vi "RT Driver VI.vi"(7 "Operation":T1, 11 "Device Reference in":T2 format="%.0x") -> (0 "Error Code":i32)   [LabVIEW 2015, in "Fuel Injection Addon Engine.lvlib"]
uses:
  Fuel Injection Addon Engine.lvlib
  <vilib>/NI Veristand/Custom Device API/Custom Device Item Ref.ctl
  <vilib>/NI Veristand/Custom Device API/Hardware Interface Driver VI Operation.ctl
  Shared/Types/Compiled.Settings.ctl
  Shared/Types/Injector info.ctl
  <vilib>/NI Veristand/Custom Device API/Waveform Data Reference.ctl
  <vilib>/NI Veristand/Custom Device API/Block Data Reference.ctl
  <vilib>/NI Veristand/Custom Device API/Data Reference.ctl
  Shared/Types/VS.Register.Info.ctl
  Shared/Types/Register.Info.ctl
  Shared/Types/FPGA Data Types.ctl
  Shared/Types/Analysis.Channels.Select.ctl
  Shared/Types/Shot.Parameters.ctl
  Shared/Types/Stage.Parameters.ctl
  Shared/Types/Stage.PullIn.Types.ctl
  Shared/Types/Stage.Transition.Types.ctl
  <vilib>/NI/NIVS Inline Async API/_VS Inline Async API/VS Inline Async API/VS Inline Async API.lvclass/VS Inline Async API.ctl
  <vilib>/NI/NIVS Inline Async API/_Data Access Engine/Data Access Engine/Data Access Engine.lvclass/Data Access Engine.ctl
  <vilib>/NI/NIVS Inline Async API/_Data Access Engine/Access Type Classes/Write/Write.lvclass/Write.ctl
  <vilib>/NI/NIVS Inline Async API/_Data Access Engine/Access Type Classes/ReadWrite/ReadWrite.lvclass/ReadWrite.ctl
  <vilib>/NI/NIVS Inline Async API/_Data Access Engine/Access Type Classes/Read/Read.lvclass/Read.ctl
  <vilib>/NI/NIVS Inline Async API/_Data Access Engine/Data Access Engine/Methods/Data.Engine.Read Data from HW.vi
  <vilib>/NI/NIVS Inline Async API/_VS Inline Async API/Error Handling Process/SubVIs/Error.GetError.vi
  <vilib>/NI/NIVS Inline Async API/_Data Access Engine/Data Access Engine/Methods/Data.Engine.Write Data to HW.vi
  <vilib>/NI/NIVS Inline Async API/_Data Access Engine/Access Type Classes/ReadWrite/ReadWrite.EngineData.vi
  <vilib>/NI/NIVS Inline Async API/_Data Access Engine/Access Type Classes/Write/Write.EngineData.vi
  <vilib>/NI/NIVS Inline Async API/_Data Access Engine/Access Type Classes/Read/Read.EngineData.vi
  <vilib>/NI Veristand/Custom Device API/NI VeriStand - Get Channel Value by Data Reference.vi
  <vilib>/NI Veristand/Custom Device API/NI VeriStand - Set Channel Value by Data Reference.vi
  <vilib>/FPGAPlugInAG/Dynamic/niLvFpga_Close_Dynamic.vi
  <vilib>/NI Veristand/Custom Device API/Global Data Refs.vi
  <vilib>/Utility/error.llb/Error Cluster From Error Code.vi
  <vilib>/rvi/errors/niLvFpgaAdjustHostInterfaceError.vi
  <vilib>/RVI Host/nirviSupport.llb/nirviErrorClusterFromErrorCode.vi
  <vilib>/Utility/config.llb/Close Config Data.vi
  <vilib>/Utility/config.llb/Write Key.vi
  <vilib>/Utility/config.llb/Write Key (I32).vi
  <vilib>/Utility/config.llb/Get Key Names.vi
  <vilib>/Utility/config.llb/Open Config Data.vi
  <vilib>/NI Veristand/Custom Device API/Get Item Property (Variant).vi
  Shared/Constants.vi
  <vilib>/rvi/interface/nirviCloseFPGA/nirviCloseFPGA.xnode
  <vilib>/rvi/interface/nirviMethod/nirviMethod.xnode
  <vilib>/NI Veristand/Custom Device Tools/Custom Device Utility Library/Custom Device Utility Library.lvlib
  <vilib>/NI/NIVS Inline Async API/_VS Inline Async API/VS Inline Async API/VS Inline Async API.lvclass
  <vilib>/rvi/interface/nirviMethod/StockFPGA_InlinedMethodWaitForSingleIRQ.vi
  <vilib>/FPGAPlugInAG/Dynamic/niLvFpga_WaitOnIrq_Dynamic.vi
  <vilib>/FPGAPlugInAG/Dynamic/niLvFpga_AcknowledgeIrq_Dynamic.vi
  <vilib>/NI VeriStand/Custom Device API/Custom Device API.lvlib
  Shared/Fuel Injection Addon Shared.lvlib
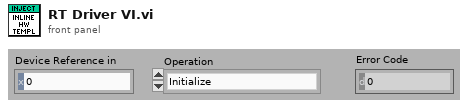
[diagram p1: front panel]
types:
  T1 = typedef "Custom Device API.lvlib/Hardware Interface Driver VI Operation.ctl" = enum16{"Initialize", "Start", "Read Data from HW", "Write Data to HW", "Close"}
  T2 = typedef "Custom Device API.lvlib/Custom Device Item Ref.ctl" = u64
  T3 = typedef "Fuel Injection Addon Engine.lvlib/Inline State Data.ctl" = cluster{"FPGA Ref":refnum<k20>, "Inline Error":errorcluster, "Sample rate (Hz)":u32, "Async":refnum<class "VS Inline Async API.lvclass">, "FPGA.Registers":T4[], "VS.Registers":T6[], "VS.Registers.Values":dbl[], "# of Registers":u32}
  T4 = typedef "Fuel Injection Addon Engine.lvlib/FPGA Refs.ctl" = cluster{"Data Type":T5, "Injector.Core.Setting":refnum<k20>, "Injector.Global.Setting":refnum<k20>, "Injector.MUX.Setting":refnum<k20>, "Index":i32, "Length":i32, "Injector.Timing":refnum<k20>}
  T5 = typedef "Fuel Injection Addon Shared.lvlib/FPGA Data Types.ctl" = enum8{"<Null>", "Injector.Core.Setting", "Injector.Global.Setting", "Injector.Mux.Setting", "Injector.Timing"}
  T6 = typedef "Custom Device API.lvlib/Block Data Reference.ctl" = cluster{"Data Reference":T7, "Offset":u64, "Length":u64}
  T7 = typedef "Custom Device API.lvlib/Data Reference.ctl" = i32
  T8 = typedef "Fuel Injection Addon Shared.lvlib/Compiled.Settings.ctl" = cluster{"Name":string, "RIO.Address":string, "Bitfile.Path":path, "Injectors.Count":u32, "Rate.Hz":u32, "Injector.Info":T9[], "Waveform.Refs":T10[], "VS.Registers":cluster{"Block Data refs":T6[], "Values":dbl[]}, "Registers":T11[], "Timing.Register":T12, "Mux.Register":T12, "Results.Selections":T13[], "Injector.Timeout":dbl, "Results.Count":i32, "Event.Parameters":T14}
  T9 = typedef "Fuel Injection Addon Shared.lvlib/Injector info.ctl" = cluster{"Results Index":i32, "Waveform Index":i32}
  T10 = typedef "Custom Device API.lvlib/Waveform Data Reference.ctl" = i32
  T11 = typedef "Fuel Injection Addon Shared.lvlib/VS.Register.Info.ctl" = cluster{"Index":i32, "Length":i32, "Register":T12}
  T12 = typedef "Fuel Injection Addon Shared.lvlib/Register.Info.ctl" = cluster{"Name":string, "Data Type":T5, "Default Value":variant}
  T13 = typedef "Fuel Injection Addon Shared.lvlib/Analysis.Channels.Select.ctl" = cluster{"Pull In Time":bool, "Pull In Max Current":bool, "Hold In Time":bool, "Hold In Max Current":bool, "Hold In Min Current":bool, "Hold In Avg Current":bool, "Hold In Avg Max Current":bool, "Hold In Avg Min Current":bool, "Hold In Max Volt":bool, "Hold In Min Volt":bool, "Hold In Avg Volt":bool, "Hold In Avg Max Volt":bool, "Hold In Avg Min Volt":bool, "Off Time":bool, "Off-Stage Max Current":bool, "Off-Stage Min Current":bool, "Off-Stage Avg Current":bool, "Total Voltage Pulses":bool}
  T14 = typedef "Fuel Injection Addon Shared.lvlib/Shot.Parameters.ctl" = cluster{"Shots":u32, "Shot.InitialVoltage":dbl, "Shot.Stages":u32, "Stages":T15[]}
  T15 = typedef "Fuel Injection Addon Shared.lvlib/Stage.Parameters.ctl" = cluster{"Stage.Dwell.Level":dbl, "PullIn.Type":T16, "PullIn.Level":dbl, "Transition.Type":T17, "Transition.Level":dbl}
  T16 = typedef "Fuel Injection Addon Shared.lvlib/Stage.PullIn.Types.ctl" = enum8{"Pull In Transition Dwells", "Pull In Transition Current Drop"}
  T17 = typedef "Fuel Injection Addon Shared.lvlib/Stage.Transition.Types.ctl" = enum8{"Stage Transition Dwell Time", "Stage Transition Voltage Level", "Stage Transition Current Drop"}
  T18 = typedef "Fuel Injection Addon Engine.lvlib/Async Parameters.ctl" = cluster{"Name":string, "Rate.Hz":u32, "Injectors.Count":u8, "Injector.Timeout":dbl, "Injector.Timer":u32[], "Injector.Info":T9[], "Events.Count":u64[], "Event.Parameters":T14, "DMA.Ref":refnum<k20>, "Waveform.Refs":T10[], "Waveform.Sessions":refnum<class "Single Waveform Write (DBL).lvclass">[], "Waveform.Enable":T19, "FPGA.Status":T20, "Search.Data":T19, "Results.Data":T20, "Results.Values":dbl[], "Results.Selections":T13[]}
  T19 = typedef "Data Access Engine.lvlib/Data Access Engine.lvclass/Read.DVR.ctl" = refnum<data-value>
  T20 = typedef "Data Access Engine.lvlib/Data Access Engine.lvclass/Write.DVR.ctl" = refnum<data-value>
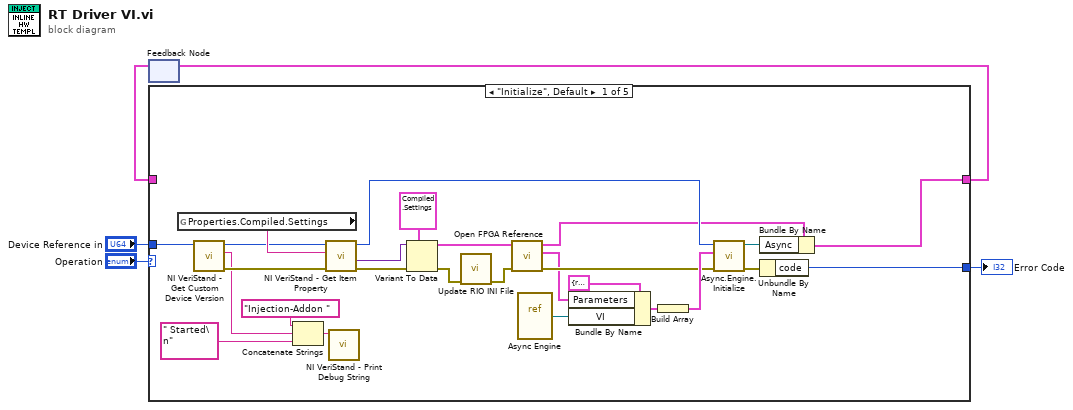
[diagram p0: block diagram]
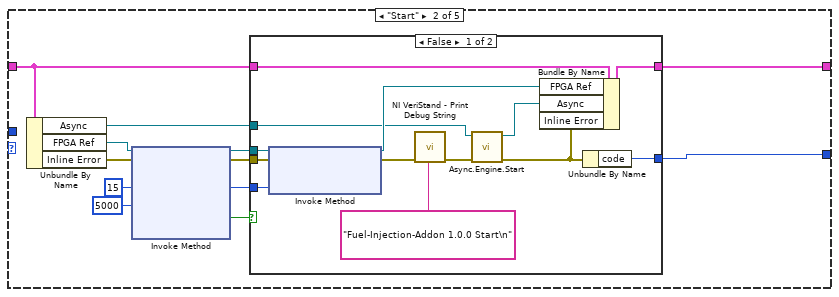
[diagram p2: hidden frame]
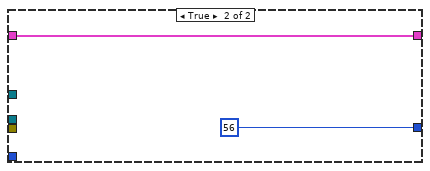
[diagram p3: hidden frame]
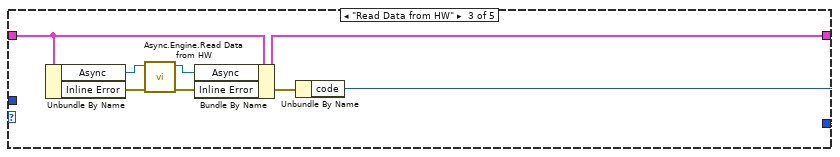
[diagram p4: hidden frame]
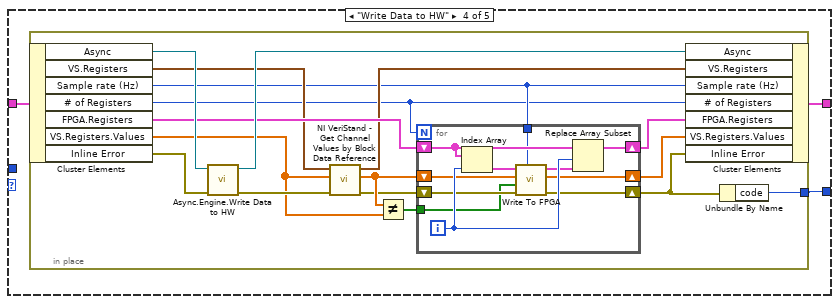
[diagram p5: hidden frame]
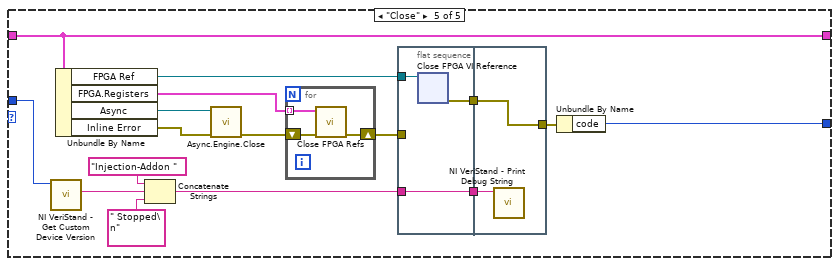
[diagram p6: hidden frame]
diagram:
  n1 = feedback #1() -> (w4:T3)  [unwired: 1 out]
  n2 = case shown="\"Initialize\", Default" "Operation" {
    tunnel: w4 -> [_ w34 w64 w67 w110]
    tunnel: "Device Reference in" -> [w11 _ _ _ w98]
    tunnel: [w31 w32 w62 w65 w101] -> w2
    tunnel: [w30 w33 w63 w66 w110] -> w1
    frame "Initialize", Default {
      n3 = global read "Constants.vi" "Properties.Compiled.Settings"() -> (w22:string)
      n4 = call <vilib>:"NI VeriStand - Get Custom Device Version.vi"("Device Ref in"=w11) -> ("error out"=w9:errorcluster, "Value"=w8:string, "Device Ref out"=w10:T2)  [unwired: 8 in]
      n5 = Concatenate Strings("Injection-Addon " ("Message"), w8, " Started\n" ("string")) -> (w28:string)
      n6 = call-poly <vilib>:"NI VeriStand - Get Item Property.vi"("error in (no error)"=w9, "Property Name"=w22, "Item Ref in"=w10) -> ("error out"=w21:errorcluster, "Value"=w20:variant, "Item Ref out"=w18:T2)  [unwired: 5 in, 1 out]
      n7 = call <vilib>:"NI VeriStand - Print Debug String.vi"("Message"=w28) -> ()  [unwired: 10 in, 1 out]
      n8 = Variant To Data(error in=w21, type=T8 {"Name"="", "RIO.Address"="", "Bitfile.Path"=path "", "Injectors.Count"=0, "Rate.Hz"=0, "Injector.Info"=[], "Waveform.Refs"=[], "VS.Registers"={"Block Data refs"=[], "Values"=[]}, "Registers"=[], "Timing.Register"={"Name"="", "Data Type"=enum."<Null>", "Default Value"=variant(dbl 0.0)}, "Mux.Register"={"Name"="", "Data Type"=enum."<Null>", "Default Value"=variant(dbl 0.0)}, "Results.Selections"=[], "Injector.Timeout"=0.0, "Results.Count"=0, "Event.Parameters"={"Shots"=0, "Shot.InitialVoltage"=0.0, "Shot.Stages"=0, "Stages"=[]}} ("Settings.Compiled"), Variant=w20) -> (data=w15:T8, error out=w13:errorcluster)
      n9 = call "Update RIO INI File.vi"("error in (no error)"=w13) -> ("error out"=w12:errorcluster)  [unwired: 10 in]
      n10 = call "Open FPGA Reference.vi"("Error In"=w12, "Settings.Compiled"=w15) -> ("Error Out"=w17:errorcluster, "Async Parameters"=w14:T18, "Inline State Data out"=w16:T3)  [unwired: 7 in]
      n11 = vi-ref "Async Engine.vi"() -> (w6:refnum<vi>)
      n12 = Bundle By Name(cluster=cluster{"VI":refnum<vi>, "Parameters":variant} {"VI"=refnum, "Parameters"=variant} ("Process"), "Parameters"=w14, "VI"=w6) -> (w26:cluster{"VI":refnum<vi>, "Parameters":variant})
      n13 = Build Array(w26) -> (w25:cluster{"VI":refnum<vi>, "Parameters":variant}[])
      n14 = call <vilib>:"Async.Engine.Initialize.vi"("error in (no error)"=w17, "Processes"=w25, "Custom Device Ref"=w18) -> ("error out"=w24:errorcluster, "Async"=w23:refnum<class "VS Inline Async API.lvclass">)  [unwired: 7 in]
      n15 = Bundle By Name(cluster=w16, "Async"=w23) -> (w30:T3)
      n16 = Unbundle By Name(w24) -> ("code"=w31:i32)
    }
    frame "Start" {
      w40 = 15 ("IRQ Number(s)")
      n17 = Unbundle By Name(w34) -> ("Async"=w35:refnum<class "VS Inline Async API.lvclass">, "FPGA Ref"=w36:refnum<k20>, "Inline Error"=w37:errorcluster)
      n18 = xnode "Invoke Method"("FPGA VI Reference In"=w36, "error in"=w37, "IRQ Number(s)"=w40, "Timeout (ms)"=5000) -> ("FPGA VI Reference Out"=w38:refnum<k20>, "error out"=w39:errorcluster, "Timed Out"=w42:bool)  [unwired: 1 out]
      n19 = case shown="False" w42 {
        tunnel: [w55 56 ("code")] -> w32
        tunnel: w34 -> [w54 w56]
        tunnel: [w53 w56] -> w33
        tunnel: w38 -> [w51 _]
        tunnel: w39 -> [w50 _]
        tunnel: w40 -> [w49 _]
        tunnel: w35 -> [w44 _]
        frame False {
          n20 = xnode "Invoke Method"("FPGA VI Reference In"=w51, "error in"=w50, "IRQ Number(s)"=w49) -> ("FPGA VI Reference Out"=w48:refnum<k20>, "error out"=w47:errorcluster)
          n21 = call <vilib>:"NI VeriStand - Print Debug String.vi"("error in (no error)"=w47, "Message"="Fuel-Injection-Addon 1.0.0 Start\n") -> ("error out"=w46:errorcluster)  [unwired: 9 in]
          n22 = call <vilib>:"Async.Engine.Start.vi"("error in (no error)"=w46, "VS Inline Async API in"=w44) -> ("error out"=w45:errorcluster, "VS Inline Async API out"=w43:refnum<class "VS Inline Async API.lvclass">)  [unwired: 8 in]
          n23 = Bundle By Name(cluster=w54, "FPGA Ref"=w48, "Async"=w43, "Inline Error"=w45) -> (w53:T3)
          n24 = Unbundle By Name(w45) -> ("code"=w55:i32)
        }
        frame True {
        }
      }
    }
    frame "Read Data from HW" {
      n25 = Unbundle By Name(w64) -> ("Async"=w60:refnum<class "VS Inline Async API.lvclass">, "Inline Error"=w61:errorcluster)
      n26 = call <vilib>:"Async.Engine.Read Data from HW.vi"("error in"=w61, "Async in"=w60) -> ("error out"=w58:errorcluster, "Async out"=w59:refnum<class "VS Inline Async API.lvclass">)  [unwired: 8 in]
      n27 = Bundle By Name(cluster=w64, "Async"=w59, "Inline Error"=w58) -> (w63:T3)
      n28 = Unbundle By Name(w58) -> ("code"=w62:i32)
    }
    frame "Write Data to HW" {
      n29 = in-place {
        in-place-border: [w68] -> w65
        n30 = in-place-cluster #2(w67) -> ("Async"=w80:refnum<class "VS Inline Async API.lvclass">, "VS.Registers"=w73:T6[], "Sample rate (Hz)"=w71:u32, "# of Registers"=w70:u32, "FPGA.Registers"=w77:T4[], "VS.Registers.Values"=w74:dbl[], "Inline Error"=w79:errorcluster)
        n31 = call <vilib>:"Async.Engine.Write Data to HW.vi"("error in (no error)"=w79, "VS Inline Async API in"=w80) -> ("error out"=w81:errorcluster, "VS Inline Async API out"=w78:refnum<class "VS Inline Async API.lvclass">)  [unwired: 8 in]
        n32 = call <vilib>:"NI VeriStand - Get Channel Values by Block Data Reference.vi"("error in (no error)"=w81, "Values Array in"=w74, "Block Data Ref"=w73) -> ("error out"=w82:errorcluster, "Values Array out"=w83:dbl[], "Block Data Ref dup"=w72:T6[])  [unwired: 6 in]
        n33 = Not Equal?(x=w83, y=w74) -> (x != y?=w84:bool[])
        n34 = for {
          N: w70 -> [_]
          shift-right: [w88] -> w75
          shift-left: w83 -> [w89]
          shift-right: [w95] -> w76
          shift-left: w77 -> [w94]
          shift-right: [w91] -> w69
          shift-left: w82 -> [w92]
          tunnel: w84 -> [w90]
          tunnel: w71 -> [w85]
          i -> [w93]
          n35 = Index Array(array=w94, index=w93) -> (element=w87:T4)
          n36 = call "Write To FPGA.vi"("Sample Rate"=w85, "error in (no error)"=w92, "Changed?"=w90, "Values"=w89, "FPGA Refs"=w87) -> ("error out"=w91:errorcluster, "Values out"=w88:dbl[], "FPGA Refs"=w86:T4)  [unwired: 4 in]
          n37 = Replace Array Subset(array=w94, new element=w86, index=w93) -> (w95:T4[])
        }
        n38 = in-place-cluster #2("Async"=w78, "VS.Registers"=w72, "Sample rate (Hz)"=w71, "# of Registers"=w70, "FPGA.Registers"=w76, "VS.Registers.Values"=w75, "Inline Error"=w69) -> (w66:T3)
        n39 = Unbundle By Name(w69) -> ("code"=w68:i32)
      }
    }
    frame "Close" {
      n40 = call <vilib>:"NI VeriStand - Get Custom Device Version.vi"("Device Ref in"=w98) -> ("Value"=w104:string)  [unwired: 8 in, 2 out]
      n41 = Unbundle By Name(w110) -> ("FPGA Ref"=w111:refnum<k20>, "FPGA.Registers"=w106:T4[], "Async"=w108:refnum<class "VS Inline Async API.lvclass">, "Inline Error"=w109:errorcluster)
      n42 = Concatenate Strings("Injection-Addon " ("Message"), w104, " Stopped\n" ("string")) -> (w97:string)
      n43 = call <vilib>:"Async.Engine.Close.vi"("error in (no error)"=w109, "Async in"=w108) -> ("error out"=w107:errorcluster)  [unwired: 8 in, 1 out]
      n44 = for {
        shift-right: [w118] -> w100
        shift-left: w107 -> [w119]
        tunnel: w106 -> [w117] mode=indexing
        n45 = call "Close FPGA Refs.vi"("error in (no error)"=w119, "FPGA Refs"=w117) -> ("error out"=w118:errorcluster)  [unwired: 9 in]
      }
      n46 = flat-sequence {
        tunnel: w111 -> [w114]
        tunnel: w100 -> [_]
        tunnel: [w113] -> w99
        tunnel: w97 -> [w112]
        tunnel: [w112] -> w96
        tunnel: [w116] -> w102
        tunnel: w99 -> [w116]
        tunnel: w96 -> [w115]
        frame #0 {
          n47 = xnode "Close FPGA VI Reference"("FPGA VI Reference In"=w114) -> ("error out"=w113:errorcluster)  [unwired: 1 in]
        }
        frame #1 {
          n48 = call <vilib>:"NI VeriStand - Print Debug String.vi"("Message"=w115) -> ()  [unwired: 10 in, 1 out]
        }
      }
      n49 = Unbundle By Name(w102) -> ("code"=w101:i32)
    }
  }
  "Error Code" <- w2
  n50 = feedback-in #1(w1) -> ()
